vi "Eyeblinker-Init.vi"(7 "Device reference":refnum<vi>, 8 "error in (no error)":errorcluster, 10 "OutputRequest event ref":T1, 11 "InputData reference":refnum<vi>) -> (0 "error out":errorcluster, 2 "OutputRequest (dup)":T1, 3 "InputData (dup)":refnum<vi>)   [LabVIEW 2015]
doc: "Initializes a valve object. Wire its reference to the \"Device reference\" input.\n\nInputData reference: create reference from Main VI\nOutputRequest event ref: get this from Rack-Init\n\nThe outputs are just duplicates to make it easier to call a bunch of Device-Init functions."
uses:
  Typedefs/Eyeblinker.ctl
  Rack/Typedefs/OutputRequest refnum.ctl
  Rack/Typedefs/OutputRequest.ctl
  Rack/Typedefs/InputData cluster.ctl
  Rack/Methods/Port drivers/DigitalInput-DataCluster.ctl
panel:
  # "(must be on same NI card)"
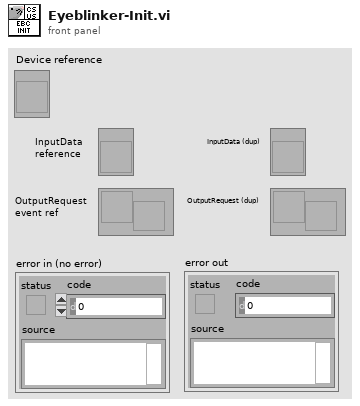
[diagram p1: front panel]
types:
  T1 = typedef "OutputRequest refnum.ctl" = refnum<user-event>
  T2 = typedef "Eyeblinker.ctl" = cluster{"Settings":cluster{"Timestamp port name":string, "Port name":string, "Port index":i32}, "OutputRequest event ref":T1, "InputData reference":refnum<vi>}
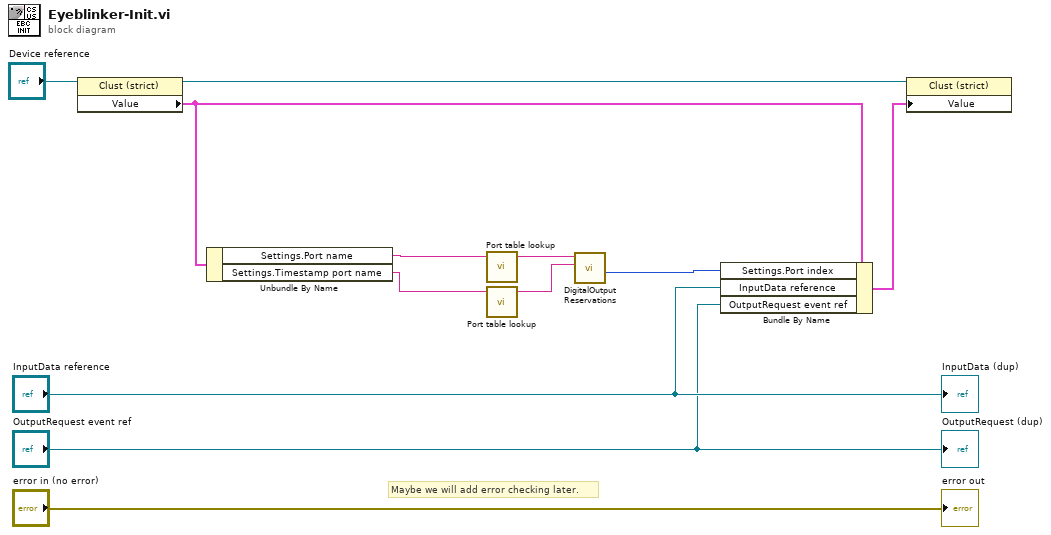
[diagram p0: block diagram]
diagram:
  # "Maybe we will add error checking later."
  n1 = property class="Clust (strict)"(reference="Device reference") -> (reference out=w5:refnum<vi>, "Value"=w7:T2)  [unwired: 1 in, 1 out]
  n2 = Unbundle By Name(w7) -> ("Settings.Port name"=w9:string, "Settings.Timestamp port name"=w10:string)
  n3 = call "Port table lookup.vi"("Port name"=w9) -> ("Line"=w11:tag)  [unwired: 3 in, 1 out]
  n4 = call "Port table lookup.vi"("Port name"=w10) -> ("Line"=w8:tag)  [unwired: 3 in, 1 out]
  n5 = call "DigitalOutput Reservations.vi"("Timestamp line"=w8, "Line"=w11) -> ("Index assigned"=w6:i32)  [unwired: 2 in, 3 out]
  n6 = Bundle By Name(cluster=w7, "Settings.Port index"=w6, "InputData reference"="InputData reference", "OutputRequest event ref"="OutputRequest event ref") -> (w4:T2)
  n7 = property class="Clust (strict)"(reference=w5, "Value"=w4) -> ()  [unwired: 1 in, 2 out]
  "error out" <- "error in (no error)"
  "OutputRequest (dup)" <- "OutputRequest event ref"
  "InputData (dup)" <- "InputData reference"
